vi "File_input_output.vi"() -> ()   [LabVIEW 2018]
panel:
  out "텍스트":string
  in  "정지 버튼":bool
  out "웨이브폼 차트":dbl(graph)
  in  "파일 경로(대화 상자 사용)":path
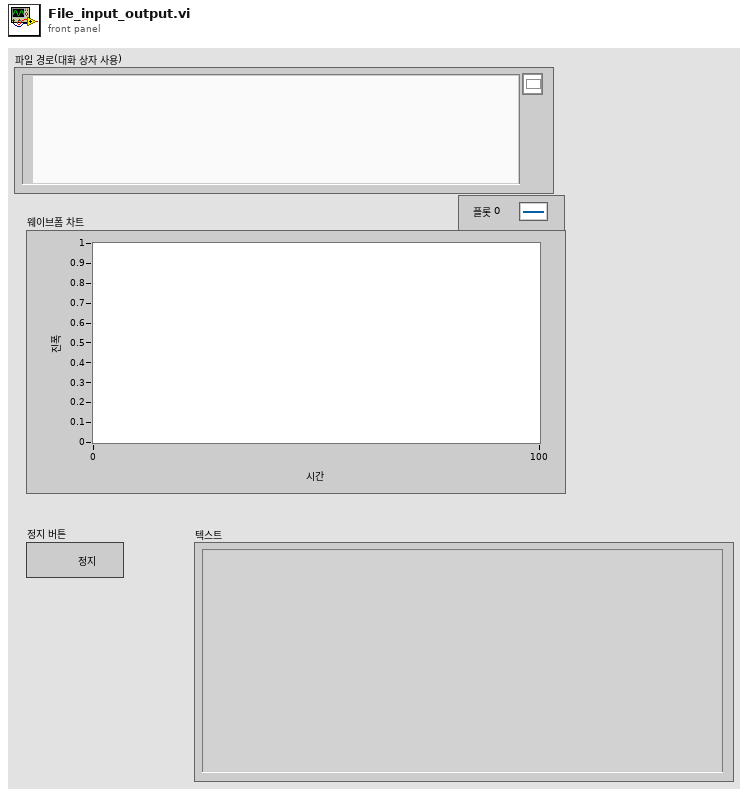
[diagram p1: front panel]
types:
  T1 = enum16{"open", "replace", "create", "open or create", "replace or create", "replace or create with confirmation"}
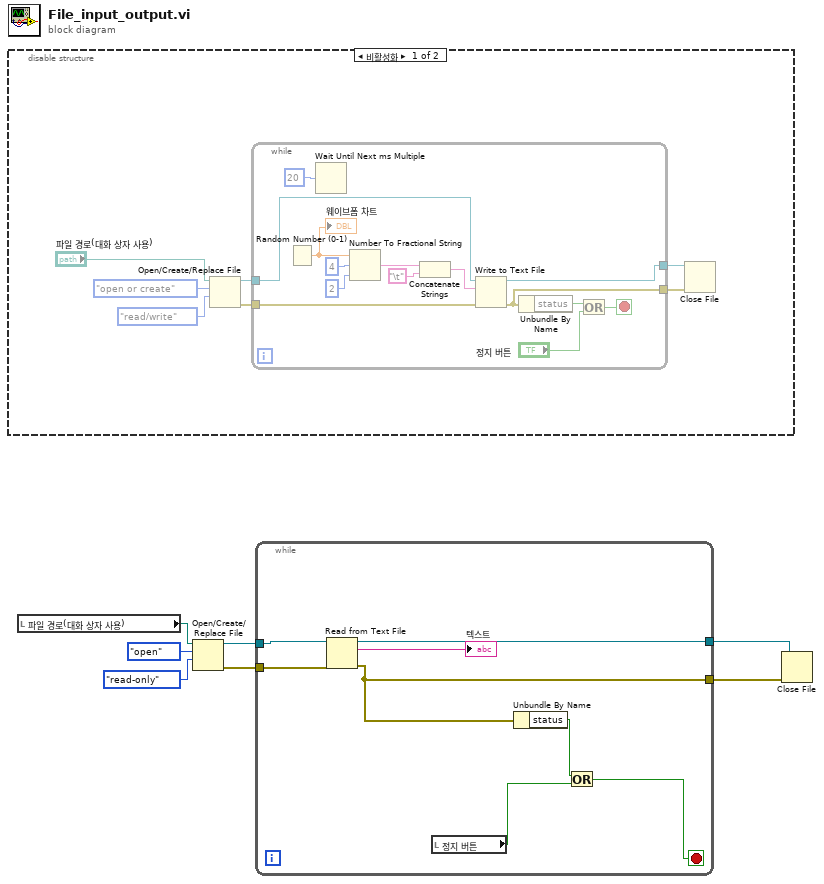
[diagram p0: block diagram]
diagram:
  n1 = disable-structure shown="비활성화" {
    frame Disabled {
      n2 = Open/Create/Replace File(file path (use dialog)="파일 경로(대화 상자 사용)", operation (0:open)=T1."open or create" ("동작(0:open)"), access (0:read/write)=enum16{"read/write", "read-only", "write-only"}."read/write" ("접근(0:읽기/쓰기)")) -> (refnum out=w11:refnum<file>, error out=w10:errorcluster)  [unwired: 3 in, 1 out]
      n3 = while {
        tunnel: w11 -> [w22]
        tunnel: w10 -> [w21]
        tunnel: [w20] -> w9
        tunnel: [w19] -> w8
        stop <- w16 stop-if-true
        n4 = Random Number (0-1)() -> (number: 0 to 1=w28:dbl)
        "웨이브폼 차트" <- w28
        n5 = Wait Until Next ms Multiple(millisecond multiple=u32 20 ("ms 배수")) -> ()  [unwired: 1 out]
        n6 = Number To Fractional String(number=w28, width (-)=i16 4 ("폭(-)"), precision (6)=i16 2 ("정밀도(6)")) -> (F-format string=w25:string)  [unwired: 1 in]
        n7 = Concatenate Strings(w25, "\t") -> (w23:string)
        n8 = Write to Text File(file (use dialog)=w22, text=w23, error in=w21) -> (refnum out=w20:refnum<file>, error out=w19:errorcluster)  [unwired: 1 in, 1 out]
        n9 = Unbundle By Name(w19) -> ("status"=w18:bool)
        n10 = Or(x=w18, y="정지 버튼") -> (x .or. y?=w16:bool)
      }
      n11 = Close File(refnum=w9, error in=w8) -> ()  [unwired: 2 out]
    }
    frame Enabled {
    }
  }
  n12 = local read "파일 경로(대화 상자 사용)"() -> (w7:path)
  n13 = Open/Create/Replace File(file path (use dialog)=w7, operation (0:open)=T1."open" ("동작(0:open)"), access (0:read/write)=enum16{"read/write", "read-only", "write-only"}."read-only" ("접근(0:읽기/쓰기)")) -> (refnum out=w4:refnum<file>, error out=w3:errorcluster)  [unwired: 3 in, 1 out]
  n14 = while {
    tunnel: w4 -> [w36]
    tunnel: w3 -> [w34]
    tunnel: [w33] -> w2
    tunnel: [w32] -> w1
    stop <- w29 stop-if-true
    n15 = Read from Text File(file (use dialog)=w36, error in=w34) -> (refnum out=w33:refnum<file>, text=→"텍스트":string, error out=w32:errorcluster)  [unwired: 2 in, 1 out]
    n16 = local read "정지 버튼"() -> (w30:bool)
    n17 = Unbundle By Name(w32) -> ("status"=w31:bool)
    n18 = Or(x=w31, y=w30) -> (x .or. y?=w29:bool)
  }
  n19 = Close File(refnum=w2, error in=w1) -> ()  [unwired: 2 out]
